vi "Read ValuesToSet(OID_TYPE_Value).vi"(8 "error in (no error)":errorcluster, 11 "RoomAlert in":refnum<class "RoomAlert.lvclass">) -> (0 "error out":errorcluster, 2 "ValuesToSet(OID/TYPE/Value)":T1=[[["1.3.6.1.4.1.20916.1.6.2.1.0", "INTEGER", "0"], ["1.3.6.1.4.1.20916.1.6.2.2.0", "INTEGER", "0"], ["1.3.6.1.4.1.20916.1.6.2.3.0", "INTEGER", "0"], ["1.3.6.1.4.1.20916.1.6.2.6.0", "INTEGER", "0"]]], 3 "RoomAlert out":refnum<class "RoomAlert.lvclass">)   [LabVIEW 2018, in "SensorPlugins.lvlib" / "RoomAlert.lvclass"]
uses:
  RoomAlert.lvclass
  TypeDefinitions/ValuesToSet.ctl
  RoomAlert.lvclass/RoomAlert.ctl
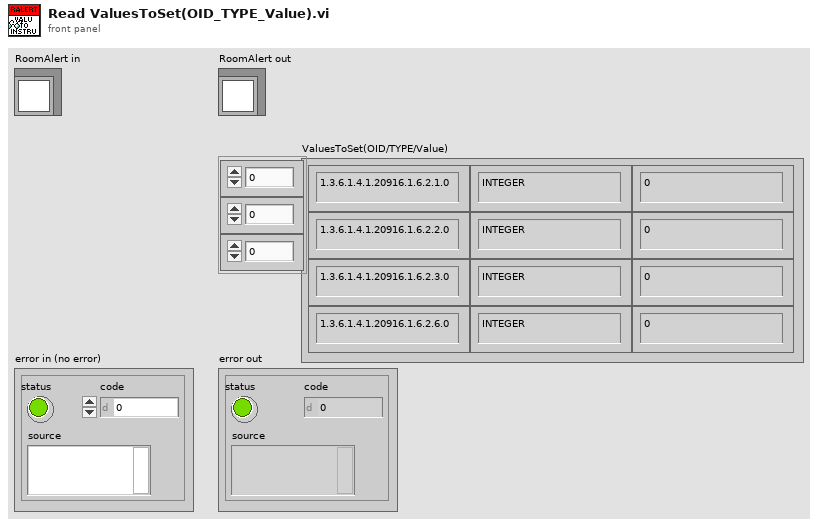
[diagram p1: front panel]
types:
  T1 = typedef "SensorPlugins.lvlib/RoomAlert.lvclass/ValuesToSet.ctl" = string[][][]
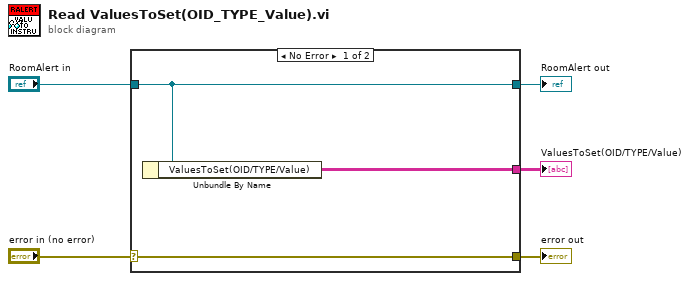
[diagram p0: block diagram]
diagram:
  n1 = case shown="No Error" "error in (no error)" {
    selector: "error in (no error)" -> [w8 w9]
    tunnel: [w8 w9] -> w4
    tunnel: [w7 w10] -> w2
    tunnel: "RoomAlert in" -> [w7 w10]
    tunnel: [w6 _] -> w1
    frame No Error {
      n2 = Unbundle By Name(w7) -> ("ValuesToSet(OID/TYPE/Value)"=w6:T1)
    }
    frame Error {
    }
  }
  "error out" <- w4
  "RoomAlert out" <- w2
  "ValuesToSet(OID/TYPE/Value)" <- w1
